vi "Show Open File Dialog (TSV CSV).vi"() -> (0 "error out":errorcluster, 3 "selected path":path)   [LabVIEW 2020]
uses:
  <vilib>/Utility/error.llb/Error Cluster From Error Code.vi
  <vilib>/ErrorRing/Error Ring.xnode
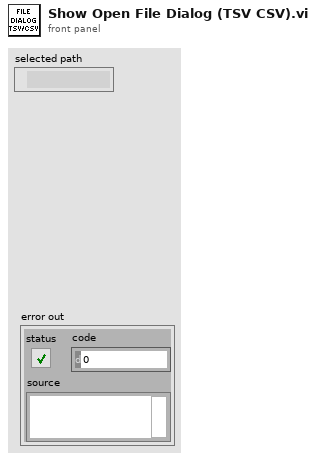
[diagram p1: front panel]
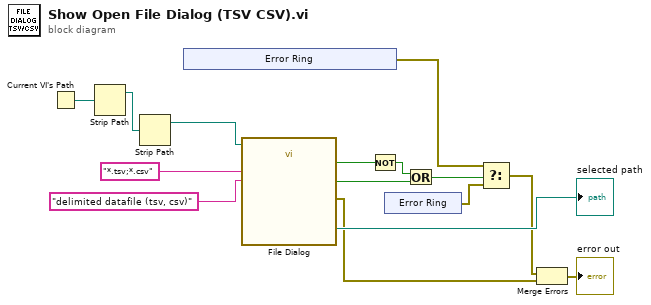
[diagram p0: block diagram]
diagram:
  n1 = Current VI's Path() -> (path=w11:path)
  n2 = Strip Path(path=w11) -> (stripped path=w12:path)  [unwired: 1 out]
  n3 = Strip Path(path=w12) -> (stripped path=w13:path)  [unwired: 1 out]
  n4 = xnode "Error Ring"() -> ("error out"=w4:errorcluster)
  n5 = call "File Dialog"("start path"=w13, "pattern (all files)"="*.tsv;*.csv", "pattern label"="delimited datafile (tsv, csv)") -> ("selected path"=→"selected path":path, "exists"=w9:bool, "cancelled"=w7:bool, "error out"=w2:errorcluster)  [unwired: 9 in]
  n6 = Not(x=w9) -> (.not. x?=w8:bool)
  n7 = xnode "Error Ring"() -> ("error out"=w5:errorcluster)
  n8 = Or(x=w8, y=w7) -> (x .or. y?=w6:bool)
  n9 = Select(t=w4, s=w6, f=w5) -> (s? t:f=w3:errorcluster)
  n10 = Merge Errors(w3, w2) -> (→"error out":errorcluster)
